vi "Login_Main P3.vi"() -> (3 "Login pass":bool)   [LabVIEW 2020]
uses:
  <vilib>/Utility/file.llb/Write Delimited Spreadsheet (string).vi
  <vilib>/Utility/file.llb/Read Delimited Spreadsheet (string).vi
  Globals/Phase III Globals.vi
panel:
  in  "Enter":bool
  in  "Stop Button":bool
  out "Pass = True":bool
  in  "Change Password":bool
  in  "Show Password":bool
  in  "Password":string
  in  "Select User":u16(ring) items=["Vigneshwaran", "Kannan"]
  # "Agnikul Cosmos"
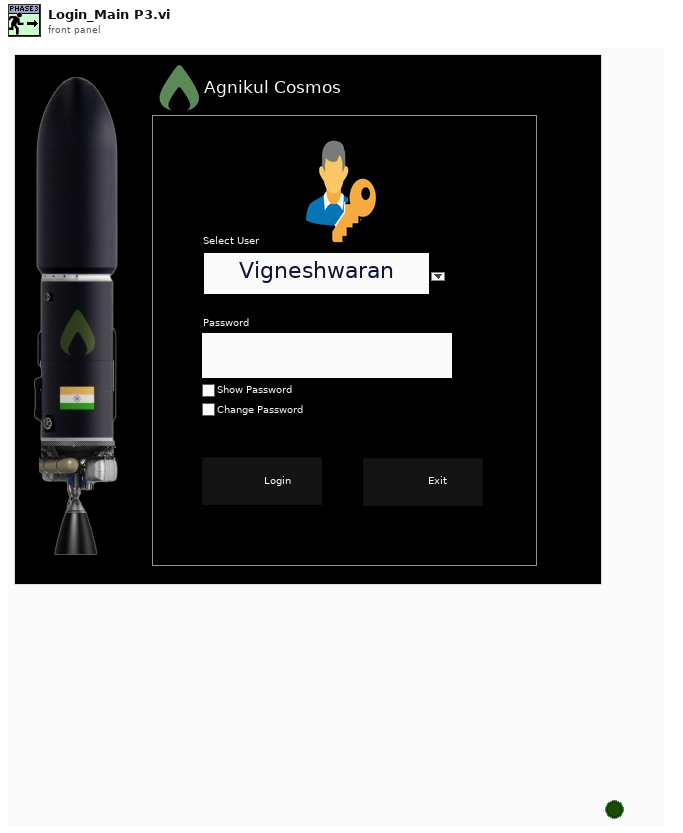
[diagram p1: front panel]
types:
  T1 = typedef "file folder ctl.ctl" = cluster{"Datalog path":path, "Configuration path":path, "Signal list path":path, "Sub vi's":path, "Authentication":path}
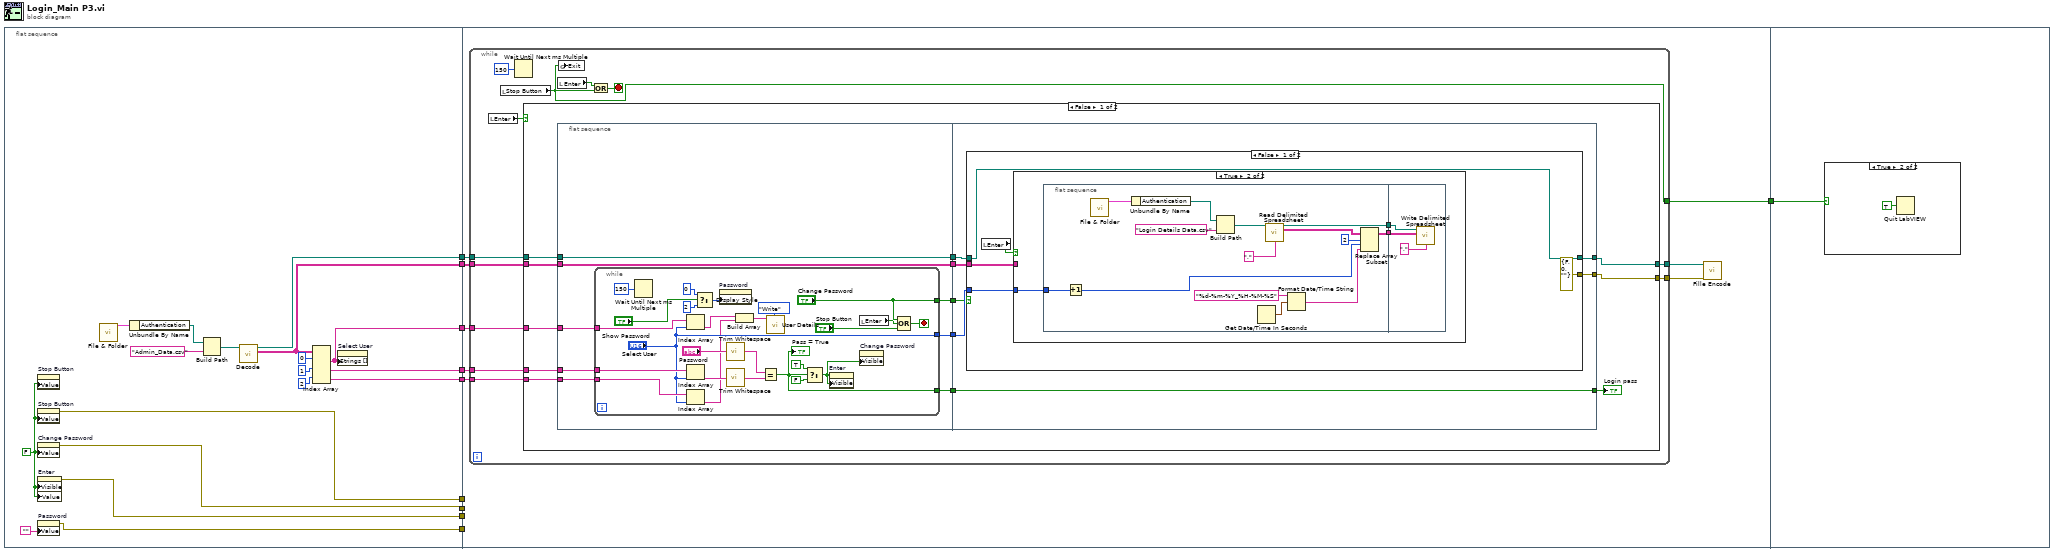
[diagram p0: block diagram]
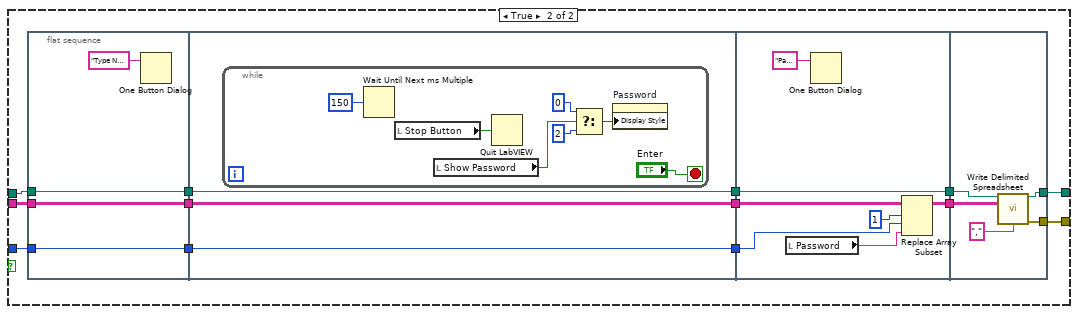
[diagram p3: hidden frame]
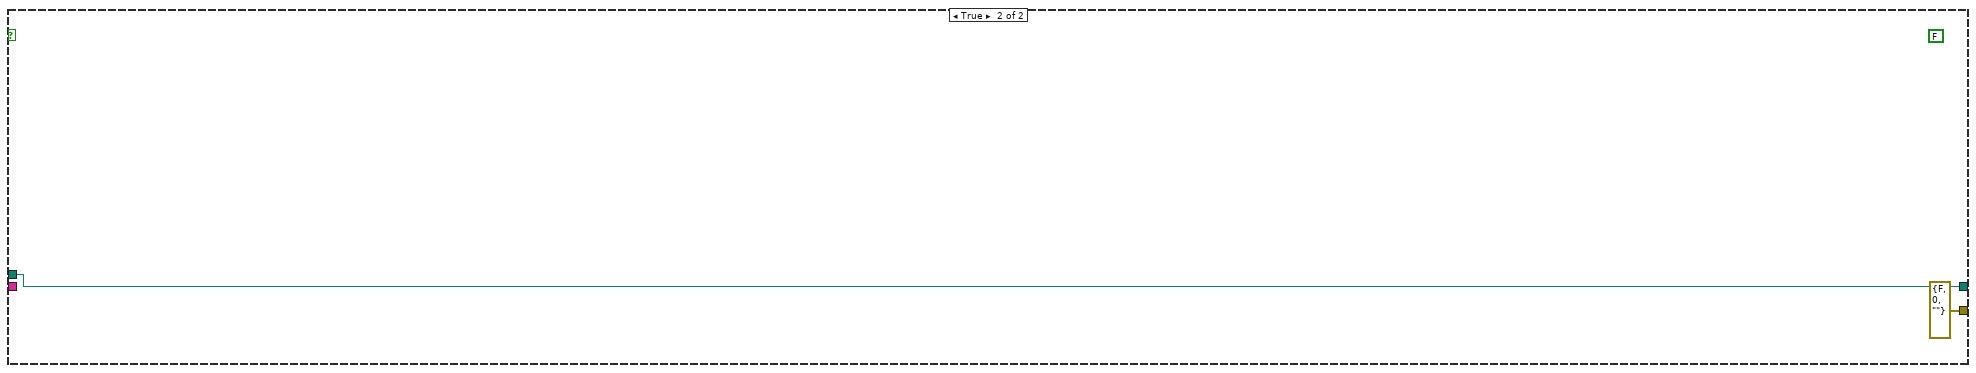
[diagram p4: hidden frame]
diagram:
  n1 = flat-sequence {
    tunnel: [w26] -> w10
    tunnel: [w11] -> w9
    tunnel: [w20] -> w8
    tunnel: [w25] -> w7
    tunnel: [w12] -> w6
    tunnel: [w22] -> w5
    tunnel: [w21] -> w4
    tunnel: [w19] -> w3
    tunnel: [w15] -> w2
    tunnel: w4 -> [_]
    tunnel: w5 -> [_]
    tunnel: w6 -> [w34]
    tunnel: w7 -> [_]
    tunnel: w8 -> [_]
    tunnel: w9 -> [w35]
    tunnel: w10 -> [w36]
    tunnel: w3 -> [w33]
    tunnel: w2 -> [w32]
    tunnel: [w31] -> w1
    tunnel: w1 -> [w168]
    frame #0 {
      w14 = FALSE ("Change Password")
      n2 = property on="Stop Button" class="Bool (strict)"("Value"=w14) -> ()  [unwired: 2 in, 2 out]
      n3 = property on="Stop Button" class="Bool (strict)"("Value"=w14) -> (error out=w21:errorcluster)  [unwired: 2 in, 1 out]
      n4 = property on="Change Password" class="Bool (strict)"("Value"=w14) -> (error out=w25:errorcluster)  [unwired: 2 in, 1 out]
      n5 = property on="Enter" class="Bool (strict)"("Visible"=w14, "Value"=w14) -> (error out=w20:errorcluster)  [unwired: 2 in, 1 out]
      n6 = property on="Password" class="Str"("Value"="") -> (error out=w22:errorcluster)  [unwired: 2 in, 1 out]
      n7 = call "File & Folder.vi"() -> ("File Output"=w18:T1)  [unwired: 10 in, 1 out]
      n8 = Unbundle By Name(w18) -> ("Authentication"=w17:path)
      n9 = Build Path(base path=w17, name or relative path="Admin_Data.csv" ("name")) -> (appended path=w13:path)
      n10 = call "Decode.vi"("Encoded  File"=w13) -> ("array"=w11:string[][], "Decoded File"=w12:path)  [unwired: 9 in]
      n11 = Index Array(array=w11, index (row) #1=0 ("index (row)"), index (row) #2=1 ("index (row)"), index (row) #3=2 ("disabled index (col)")) -> (element #1=w19:string[], element #2=w26:string[], element #3=w15:string[])  [unwired: 3 in]
      n12 = property on="Select User" class="Ring (strict)"("Strings []"=w19) -> ()  [unwired: 2 in, 2 out]
    }
    frame #1 {
      n13 = while {
        tunnel: w36 -> [w47]
        tunnel: w35 -> [w46]
        tunnel: w34 -> [w45]
        tunnel: w33 -> [w43]
        tunnel: w32 -> [w42]
        tunnel: [w39] -> w31
        tunnel: [w38] -> w30
        tunnel: [w37] -> w29
        stop <- w41 stop-if-true
        n14 = local read "Enter"() -> (w44:bool)
        n15 = local read "Stop Button"() -> (w39:bool)
        n16 = Wait Until Next ms Multiple(millisecond multiple=u32 150) -> ()  [unwired: 1 out]
        n17 = case shown="False" w44 {
          tunnel: w47 -> [w59 _]
          tunnel: w46 -> [w58 _]
          tunnel: w45 -> [w55 w167]
          tunnel: w43 -> [w54 _]
          tunnel: w42 -> [w53 _]
          tunnel: [w50 errorcluster {"status"=FALSE, "code"=0, "source"=""} ("error out")] -> w38
          tunnel: [w49 w167] -> w37
          frame False {
            n18 = flat-sequence {
              tunnel: [w69] -> w61
              tunnel: [w68] -> w60
              tunnel: w58 -> [w69]
              tunnel: w59 -> [w67]
              tunnel: [w66] -> w57
              tunnel: [w65] -> w56
              tunnel: w55 -> [w65]
              tunnel: w54 -> [w64]
              tunnel: w53 -> [w63]
              tunnel: [w62] -> w52
              tunnel: w61 -> [w101]
              tunnel: w60 -> [w100]
              tunnel: w57 -> [w99]
              tunnel: w56 -> [w95]
              tunnel: w52 -> [w98]
              tunnel: [w98] -> w51
              tunnel: [w97] -> w49
              tunnel: [w96] -> w50
              frame #0 {
                n19 = while {
                  tunnel: ["Select User"] -> w68
                  tunnel: w67 -> [w94]
                  tunnel: ["Change Password"] -> w66
                  tunnel: w64 -> [w78]
                  tunnel: w63 -> [w77]
                  tunnel: [w74] -> w62
                  stop <- w83 stop-if-true
                  n20 = Wait Until Next ms Multiple(millisecond multiple=u32 150) -> ()  [unwired: 1 out]
                  n21 = Index Array(array=w78, index="Select User") -> (element=w72:string)
                  n22 = Index Array(array=w94, index="Select User") -> (element=w93:string)
                  n23 = Index Array(array=w77, index="Select User") -> (element=w71:string)
                  n24 = Select(t=u32 0 ("Display Style"), s="Show Password", f=u32 2 ("Display Style")) -> (s? t:f=w87:u32)
                  n25 = property on="Password" class="Str"("Display Style"=w87) -> ()  [unwired: 2 in, 2 out]
                  n26 = call <vilib>:"Trim Whitespace.vi"("string"="Password") -> ("trimmed string"=w89:string)  [unwired: 1 in]
                  n27 = call <vilib>:"Trim Whitespace.vi"("string"=w93) -> ("trimmed string"=w79:string)  [unwired: 1 in]
                  n28 = Build Array(w72, w71) -> (w70:string[])
                  n29 = Equal?(x=w89, y=w79) -> (x = y?=w74:bool)
                  "Pass = True" <- w74
                  n30 = call "User Details.vi"("Enum"=enum16{"Read", "Write"}."Write", "User details"=w70) -> ()  [unwired: 8 in, 2 out]
                  n31 = Select(t=TRUE, s=w74, f=FALSE ("Visible")) -> (s? t:f=w80:bool)
                  n32 = property on="Enter" class="Bool (strict)"("Visible"=w80) -> ()  [unwired: 2 in, 2 out]
                  n33 = local read "Enter"() -> (w81:bool)
                  n34 = property on="Change Password" class="Bool (strict)"("Visible"=w80) -> ()  [unwired: 2 in, 2 out]
                  n35 = Compound Arithmetic op=OR("Change Password", w81, "Stop Button") -> (w83:bool)
                }
              }
              frame #1 {
                n36 = case shown="False" w99 {
                  tunnel: w101 -> [w106 w137]
                  tunnel: w100 -> [w105 w134]
                  tunnel: w95 -> [w103 w129]
                  tunnel: [w103 w128] -> w97
                  tunnel: [errorcluster {"status"=FALSE, "code"=0, "source"=""} ("error out") w127] -> w96
                  frame False {
                    n37 = local read "Enter"() -> (w104:bool)
                    n38 = case shown="True" w104 {
                      tunnel: w106 -> [_ _]
                      tunnel: w105 -> [_ w109]
                      frame False {
                      }
                      frame True {
                        n39 = flat-sequence {
                          tunnel: w109 -> [w123]
                          tunnel: [w113] -> w108
                          tunnel: [w112] -> w107
                          tunnel: w108 -> [w125]
                          tunnel: w107 -> [w126]
                          frame #0 {
                            n40 = Increment(x=w123) -> (x+1=w116:u16)
                            n41 = call "File & Folder.vi"() -> ("File Output"=w119:T1)  [unwired: 10 in, 1 out]
                            n42 = Unbundle By Name(w119) -> ("Authentication"=w118:path)
                            n43 = Build Path(base path=w118, name or relative path="Login Details Data.csv" ("name")) -> (appended path=w115:path)
                            n44 = Get Date/Time In Seconds() -> (seconds since 1Jan1904=w110:timestamp)
                            n45 = call-poly <vilib>:"Read Delimited Spreadsheet.vi"("file path (dialog if empty)"=w115, "delimiter (\\t)"="," ("delimiter (\\t)")) -> ("new file path (Not A Path if cancelled)"=w112:path, "all rows"=w114:string[][])  [unwired: 8 in, 4 out]
                            n46 = Format Date/Time String(time format string (%c)="%d-%m-%Y_%H-%M-%S", seconds (now)=w110) -> (date/time string=w121:string)  [unwired: 1 in]
                            n47 = Replace Array Subset(array=w114, new element=w121, index (row)=2, index (col)=w116) -> (w113:string[][])
                          }
                          frame #1 {
                            n48 = call-poly <vilib>:"Write Delimited Spreadsheet.vi"("file path (dialog if empty)"=w126, "2D data"=w125, "delimiter (\\t)"="," ("delimiter (\\t)")) -> ()  [unwired: 11 in, 2 out]
                          }
                        }
                      }
                    }
                  }
                  frame True {
                    n49 = flat-sequence {
                      tunnel: [w143] -> w138
                      tunnel: w137 -> [w143]
                      tunnel: [w142] -> w135
                      tunnel: w134 -> [w142]
                      tunnel: [w141] -> w130
                      tunnel: w129 -> [w141]
                      tunnel: [w146] -> w139
                      tunnel: w138 -> [w146]
                      tunnel: [w145] -> w136
                      tunnel: w135 -> [w145]
                      tunnel: [w144] -> w131
                      tunnel: w130 -> [w144]
                      tunnel: w139 -> [w159]
                      tunnel: w136 -> [w157]
                      tunnel: [w155] -> w133
                      tunnel: [w154] -> w132
                      tunnel: w131 -> [w154]
                      tunnel: w133 -> [w165]
                      tunnel: w132 -> [w164]
                      tunnel: [w162] -> w128
                      tunnel: [w161] -> w127
                      frame #0 {
                        n50 = One Button Dialog(message="Type New Password and Press Enter button") -> ()  [unwired: 1 in, 1 out]
                      }
                      frame #1 {
                        n51 = while {
                          stop <- "Enter" stop-if-true
                          n52 = Wait Until Next ms Multiple(millisecond multiple=u32 150) -> ()  [unwired: 1 out]
                          n53 = local read "Stop Button"() -> (w152:bool)
                          n54 = local read "Show Password"() -> (w147:bool)
                          n55 = Quit LabVIEW(quit? (T)=w152) -> ()
                          n56 = Select(t=u32 0 ("Display Style"), s=w147, f=u32 2 ("Display Style")) -> (s? t:f=w148:u32)
                          n57 = property on="Password" class="Str"("Display Style"=w148) -> ()  [unwired: 2 in, 2 out]
                        }
                      }
                      frame #2 {
                        n58 = local read "Password"() -> (w156:string)
                        n59 = One Button Dialog(message="Password changed successfully, Please Login with new Password") -> ()  [unwired: 1 in, 1 out]
                        n60 = Replace Array Subset(array=w159, new element=w156, index (row)=1, index (col)=w157) -> (w155:string[][])
                      }
                      frame #3 {
                        n61 = call-poly <vilib>:"Write Delimited Spreadsheet.vi"("file path (dialog if empty)"=w164, "2D data"=w165, "delimiter (\\t)"="," ("delimiter (\\t)")) -> ("new file path (Not A Path if cancelled)"=w162:path, "error out"=w161:errorcluster)  [unwired: 11 in]
                      }
                    }
                  }
                }
              }
            }
            "Login pass" <- w51
          }
          frame True {
            (unwired) FALSE
          }
        }
        n62 = local read "Enter"() -> (w40:bool)
        n63 = global write "Phase III Globals.vi" "Exit"(w39) -> ()
        n64 = Compound Arithmetic op=OR(w40, w39) -> (w41:bool)
      }
      n65 = call "Fille Encode.vi"("error in"=w30, "Original File"=w29) -> ()  [unwired: 8 in, 2 out]
    }
    frame #2 {
      n66 = case shown="True" w168 {
        frame False {
        }
        frame True {
          n67 = Quit LabVIEW(quit? (T)=TRUE) -> ()
        }
      }
    }
  }
